vi "Homing_Modbus.vi"(0 "Modbus master in":refnum<class "Modbus Master.lvclass">, 1 "Homing Timeout":u16, 2 "Prehoming Position":u16[](array[numeric]), 3 "Prehoming Hardware Torque":u16, 4 "Prehoming Software Torque":u16, 5 "Homing Position":u16[](array[numeric]), 6 "Homing Hardware Torque":u16, 7 "error in (no error)":errorcluster, 8 "Homing Parameters":cluster{"Home":bool, "Start":bool}, 9 "Homing Software Torque":u16) -> (20 "Modbus master out":refnum<class "Modbus Master.lvclass">, 27 "error out":errorcluster)   [LabVIEW 2021]
uses:
  <vilib>/Modbus/master/Modbus Master.lvclass
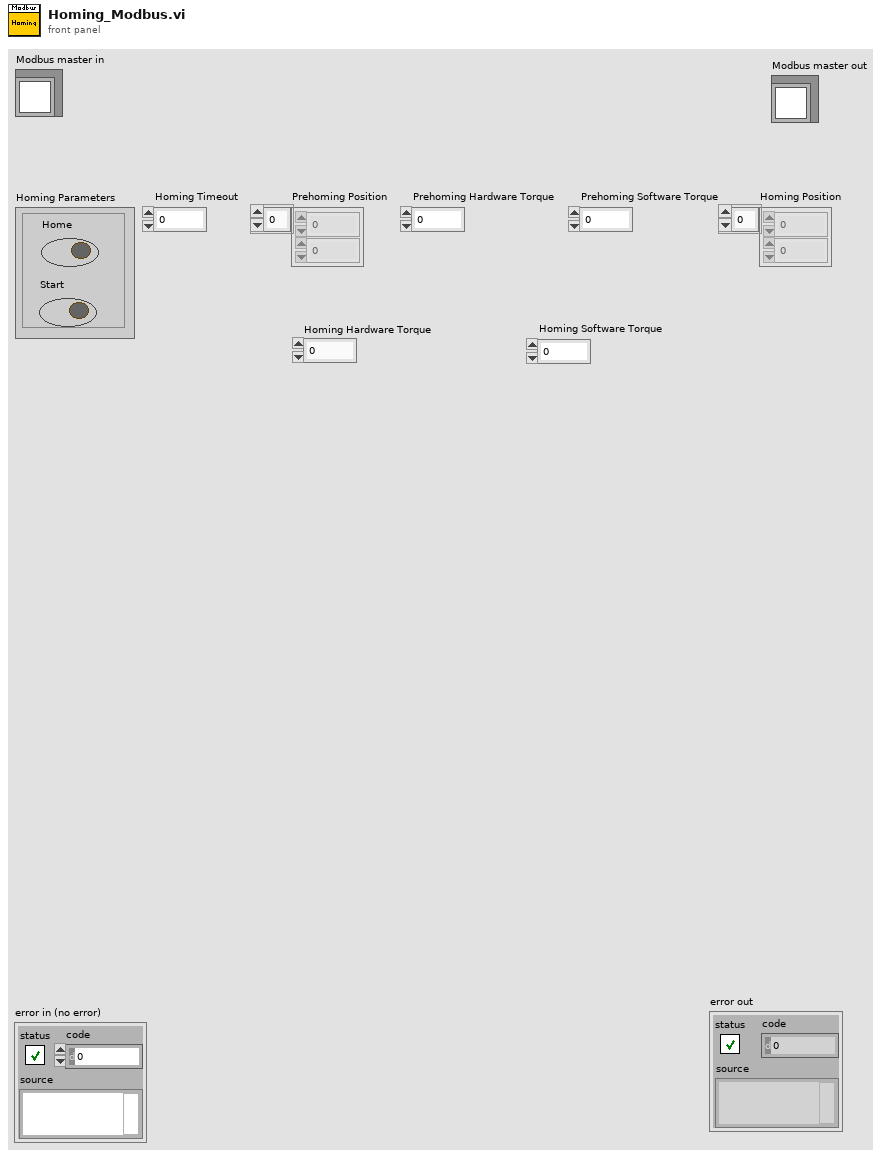
[diagram p1: front panel]
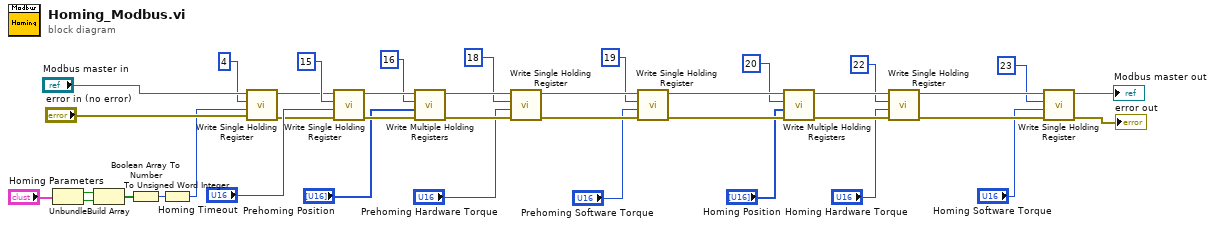
[diagram p0: block diagram]
diagram:
  n1 = Unbundle("Homing Parameters") -> ("Home"=w35:bool, "Start"=w36:bool)
  n2 = Build Array(w35, w36) -> (w34:bool[])
  n3 = Boolean Array To Number(Boolean array=w34) -> (number=w33:u32)
  n4 = To Unsigned Word Integer(number=w33) -> (unsigned 16bit integer=w32:u16)
  n5 = call-dynamic "Write Single Holding Register.vi"("error in (no error)"="error in (no error)", "holding register value"=w32, "address"=u16 4, "Modbus master in"="Modbus master in") -> ("error out"=w26:errorcluster, "Modbus master out"=w28:refnum<class "Modbus Master.lvclass">)  [unwired: 6 in]
  n6 = call-dynamic "Write Single Holding Register.vi"("error in (no error)"=w26, "holding register value"="Homing Timeout", "address"=u16 15, "Modbus master in"=w28) -> ("error out"=w25:errorcluster, "Modbus master out"=w27:refnum<class "Modbus Master.lvclass">)  [unwired: 6 in]
  n7 = call-dynamic "Write Multiple Holding Registers.vi"("error in (no error)"=w25, "holding register values"="Prehoming Position", "starting address"=u16 16, "Modbus master in"=w27) -> ("error out"=w22:errorcluster, "Modbus master out"=w21:refnum<class "Modbus Master.lvclass">)  [unwired: 6 in]
  n8 = call-dynamic "Write Single Holding Register.vi"("error in (no error)"=w22, "holding register value"="Prehoming Hardware Torque", "address"=u16 18, "Modbus master in"=w21) -> ("error out"=w18:errorcluster, "Modbus master out"=w17:refnum<class "Modbus Master.lvclass">)  [unwired: 6 in]
  n9 = call-dynamic "Write Single Holding Register.vi"("error in (no error)"=w18, "holding register value"="Prehoming Software Torque", "address"=u16 19, "Modbus master in"=w17) -> ("error out"=w14:errorcluster, "Modbus master out"=w13:refnum<class "Modbus Master.lvclass">)  [unwired: 6 in]
  n10 = call-dynamic "Write Multiple Holding Registers.vi"("error in (no error)"=w14, "holding register values"="Homing Position", "starting address"=u16 20, "Modbus master in"=w13) -> ("error out"=w9:errorcluster, "Modbus master out"=w10:refnum<class "Modbus Master.lvclass">)  [unwired: 6 in]
  n11 = call-dynamic "Write Single Holding Register.vi"("error in (no error)"=w9, "holding register value"="Homing Hardware Torque", "address"=u16 22, "Modbus master in"=w10) -> ("error out"=w7:errorcluster, "Modbus master out"=w8:refnum<class "Modbus Master.lvclass">)  [unwired: 6 in]
  n12 = call-dynamic "Write Single Holding Register.vi"("error in (no error)"=w7, "holding register value"="Homing Software Torque", "address"=u16 23, "Modbus master in"=w8) -> ("error out"=→"error out":errorcluster, "Modbus master out"=→"Modbus master out":refnum<class "Modbus Master.lvclass">)  [unwired: 6 in]
